vi "HP81110A Output Set - Fast.vi"(6 "notoutput2":bool caption="Not-Output 2", 7 "output1":bool caption="Output 1", 8 "error in (no error)":errorcluster, 9 "output2":bool caption="Output 2", 10 "notoutput1":bool caption="Not-Output 1", 11 "VISA session":refnum<visa-resource-name>) -> (0 "error out":errorcluster, 3 "dup VISA session":refnum<visa-resource-name>)   [LabVIEW 2015]
doc: "This behaves just like the \"Output Set\" function, except it issues all four commands at once instead of as four separate commands with model queries in between. The result: the outputs turn on/off visibly faster. The difference is especially noticeable when you turn all four on at once, or all four off at once."
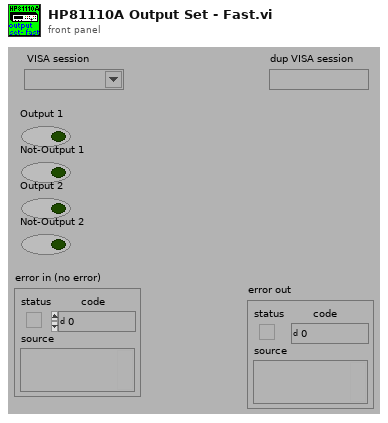
[diagram p1: front panel]
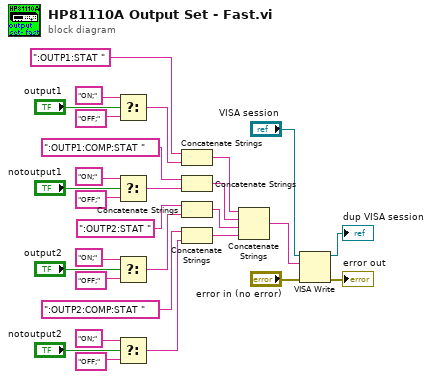
[diagram p0: block diagram]
diagram:
  n1 = Select(t="ON;", s="output1", f="OFF;") -> (s? t:f=w20:string)
  n2 = Select(t="ON;", s="notoutput1", f="OFF;") -> (s? t:f=w16:string)
  n3 = Select(t="ON;", s="output2", f="OFF;") -> (s? t:f=w13:string)
  n4 = Select(t="ON;", s="notoutput2", f="OFF;") -> (s? t:f=w10:string)
  n5 = Concatenate Strings(":OUTP1:STAT ", w20) -> (w9:string)
  n6 = Concatenate Strings(":OUTP1:COMP:STAT ", w16) -> (w8:string)
  n7 = Concatenate Strings(":OUTP2:STAT ", w13) -> (w7:string)
  n8 = Concatenate Strings(":OUTP2:COMP:STAT ", w10) -> (w6:string)
  n9 = Concatenate Strings(w9, w8, w7, w6) -> (w3:string)
  n10 = VISA Write(VISA resource name="VISA session", write buffer=w3, error in (no error)="error in (no error)") -> (VISA resource name out=→"dup VISA session":refnum<visa-resource-name>, error out=→"error out":errorcluster)  [unwired: 1 out]
